vi "Read Refnum String.vi"(8 "error in (no error)":errorcluster, 11 "Arithmetic_Operations in":refnum<class "Arithmetic_Operations.lvclass">) -> (0 "error out":errorcluster, 2 "Refnum String":string, 3 "Arithmetic_Operations out":refnum<class "Arithmetic_Operations.lvclass">)   [LabVIEW 2020, in "Arithmetic_Operations.lvclass"]
uses:
  Arithmetic_Operations.lvclass
  Arithmetic_Operations.lvclass/Arithmetic_Operations.ctl
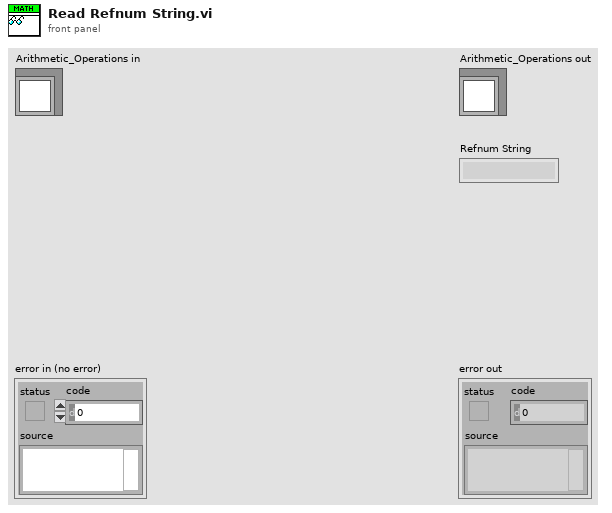
[diagram p1: front panel]
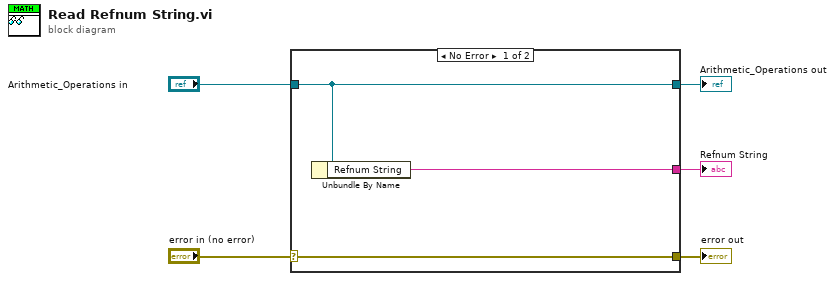
[diagram p0: block diagram]
diagram:
  n1 = case shown="No Error" "error in (no error)" {
    selector: "error in (no error)" -> [w8 w9]
    tunnel: [w8 w9] -> w4
    tunnel: [w7 w10] -> w2
    tunnel: "Arithmetic_Operations in" -> [w7 w10]
    tunnel: [w6 _] -> w1
    frame No Error {
      n2 = Unbundle By Name(w7) -> ("Refnum String"=w6:string)
    }
    frame Error {
    }
  }
  "error out" <- w4
  "Arithmetic_Operations out" <- w2
  "Refnum String" <- w1
